vi "KrakenCommandVelocity.vi"(0 "Device Reference (in)":T1, 5 "Output Mode":T2(ring), 7 "Control Mode":enum16{"Safety", "Power", "Velocity"}(ring), 9 "Power or Testing Power":dbl, 11 "Error (in)":errorcluster) -> (4 "Device Reference (out)":T1, 15 "Error (out)":errorcluster)   [LabVIEW 2023]
doc: "Wrapper for commanding the power of a Talon FX motor controller. Supports voltage and safety interlock. Also supports the standard actuator testing interface and and the only sending new values on change."
uses:
  <vilib>/Rock Robotics/WPI/ThirdParty/Phoenix6/DeviceReference.ctl
  <vilib>/Rock Robotics/WPI/ThirdParty/Phoenix6/controls/DutyCycleOut SetControl.vi
  <vilib>/Rock Robotics/WPI/ThirdParty/Phoenix6/controls/VelocityDutyCycle SetControl.vi
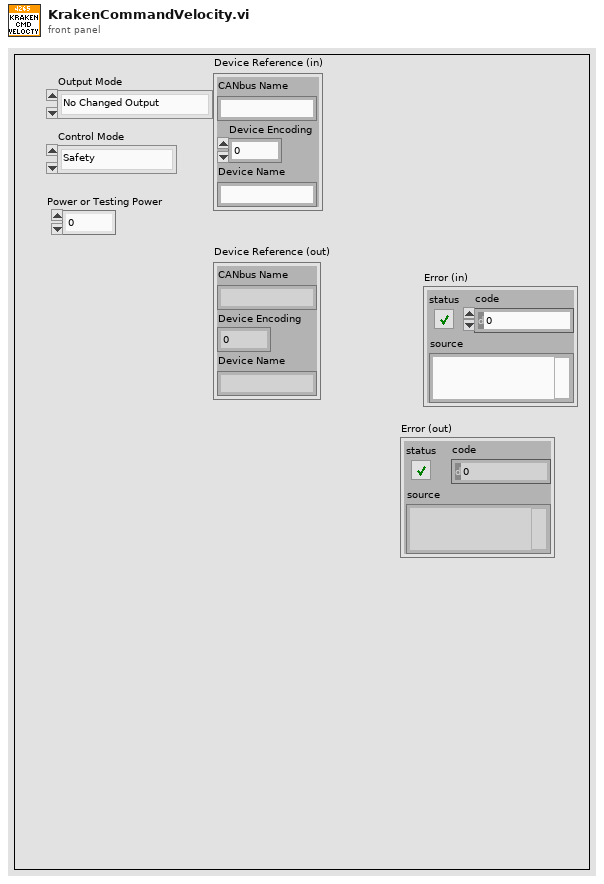
[diagram p1: front panel]
types:
  T1 = typedef "DeviceReference.ctl" = cluster{"CANbus Name":string, "Device Encoding":u32, "Device Name":string}
  T2 = enum16{"No Changed Output", "New Normal Output", "New Testing Output"}
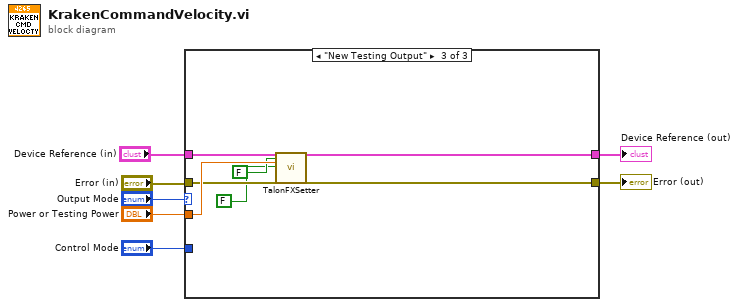
[diagram p0: block diagram]
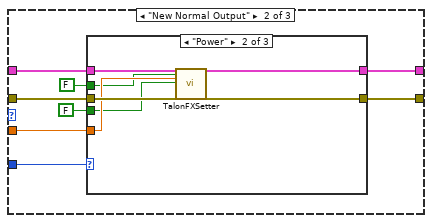
[diagram p3: hidden frame]
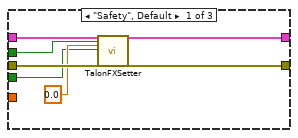
[diagram p4: hidden frame]
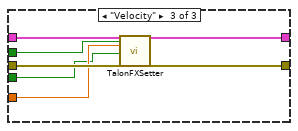
[diagram p5: hidden frame]
diagram:
  n1 = case shown="\"New Testing Output\"" "Output Mode" {
    tunnel: "Power or Testing Power" -> [_ w14 w45]
    tunnel: "Device Reference (in)" -> [w9 w17 w43]
    tunnel: "Control Mode" -> [_ w16 _]
    tunnel: "Error (in)" -> [w8 w15 w44]
    tunnel: [w9 w12 w41] -> w2
    tunnel: [w8 w11 w40] -> w1
    frame "No Changed Output", Default {
    }
    frame "New Normal Output" {
      n2 = case shown="\"Power\"" w16 {
        tunnel: w17 -> [w23 w31 w38]
        tunnel: w14 -> [_ w29 w35]
        tunnel: w15 -> [w24 w30 w37]
        tunnel: FALSE ("StopSendingOtherRequests") -> [w21 w28 w36]
        tunnel: [w20 w27 w34] -> w12
        tunnel: [w19 w26 w33] -> w11
        tunnel: FALSE ("EnableFOC") -> [w18 w25 w32]
        frame "Safety", Default {
          n3 = call-poly <vilib>:"TalonFXSetter.vi"("DeviceReference"=w23, "StopSendingOtherRequests"=w21, "Output"=0.0, "EnableFOC"=w18, "error in"=w24) -> ("DeviceReference Out"=w20:T1, "error out"=w19:errorcluster)  [unwired: 21 in]
        }
        frame "Power" {
          n4 = call-poly <vilib>:"TalonFXSetter.vi"("DeviceReference"=w31, "StopSendingOtherRequests"=w28, "Output"=w29, "EnableFOC"=w25, "error in"=w30) -> ("DeviceReference Out"=w27:T1, "error out"=w26:errorcluster)  [unwired: 21 in]
        }
        frame "Velocity" {
          n5 = call-poly <vilib>:"TalonFXSetter.vi"("DeviceReference"=w38, "StopSendingOtherRequests"=w36, "Velocity"=w35, "EnableFOC"=w32, "error in"=w37) -> ("DeviceReference Out"=w34:T1, "error out"=w33:errorcluster)  [unwired: 21 in]
        }
      }
    }
    frame "New Testing Output" {
      n6 = call-poly <vilib>:"TalonFXSetter.vi"("DeviceReference"=w43, "StopSendingOtherRequests"=FALSE, "Output"=w45, "EnableFOC"=FALSE, "error in"=w44) -> ("DeviceReference Out"=w41:T1, "error out"=w40:errorcluster)  [unwired: 21 in]
    }
  }
  "Device Reference (out)" <- w2
  "Error (out)" <- w1
